vi "Builder.Get Builder Status.vi"(11 "Builder in":refnum<class "Builder.lvclass">) -> (2 "Builder Status":refnum<class "Builder Status.lvclass">, 3 "Builder out":refnum<class "Builder.lvclass">)   [LabVIEW 2016, in "DSF.Engine.lvlib" / "Builder.lvclass"]
uses:
  Builder.lvclass
  Status/Builder Status.lvclass
  Builder.lvclass/Builder.ctl
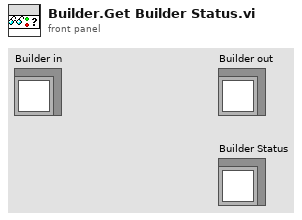
[diagram p1: front panel]
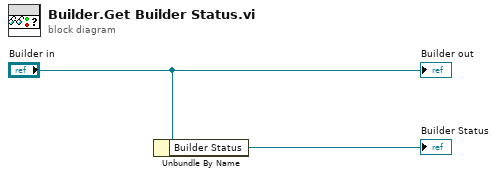
[diagram p0: block diagram]
diagram:
  n1 = Unbundle By Name("Builder in") -> ("Builder Status"=→"Builder Status":refnum<class "Builder Status.lvclass">)
  "Builder out" <- "Builder in"
